vi "solar_msg Q Name.vi"(0 "Queue":refnum<queue>) -> (5 "Valid Queue?":bool, 6 "Queue Name":string)   [LabVIEW 2018]
doc: "This returns the queue name"
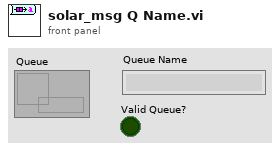
[diagram p1: front panel]
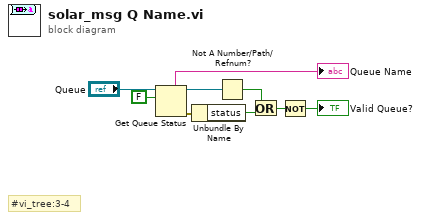
[diagram p0: block diagram]
diagram:
  # "#vi_tree:3-4"
  n1 = Get Queue Status(queue="Queue", return elements? (F)=FALSE ("Return Elements (F)")) -> (queue out=w2:refnum<queue>, queue name=→"Queue Name":string, error out=w9:errorcluster)  [unwired: 1 in, 5 out]
  n2 = Unbundle By Name(w9) -> ("status"=w8:bool)
  n3 = Not A Number/Path/Refnum?(number/path/refnum=w2) -> (NaN/Path/Refnum?=w6:bool)
  n4 = Or(x=w6, y=w8) -> (x .or. y?=w5:bool)
  n5 = Not(x=w5) -> (.not. x?=→"Valid Queue?":bool)
